vi "Tool Test Tool Test.vi"   [LabVIEW 2019]
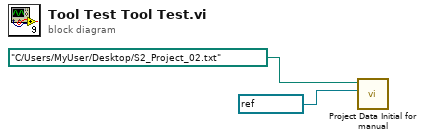
[diagram p0: block diagram]
diagram:
  n1 = call "Project Data Initial for manual.vi"("VISA resource name"=refnum<visa-resource-name> "COM2", "configuration file path"=path "C:/Users/MyUser/Desktop/S2_Project_02.txt") -> ()  [unwired: 6 in, 4 out]
